vi "Load State.vi"(8 "error in":errorcluster, 11 "State File Refnum":refnum<file>) -> (0 "error out":errorcluster, 1 "Out-of-range List":string[](array[string]), 2 "Monitoring List":string[](array[string]), 3 "refnum out":refnum<file>)   [LabVIEW 2013, in "ACNET Monitor.lvlib"]
uses:
  ACNET Monitor.lvlib
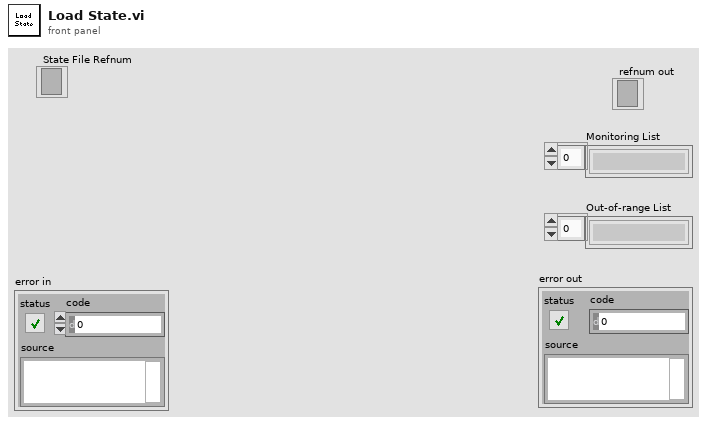
[diagram p1: front panel]
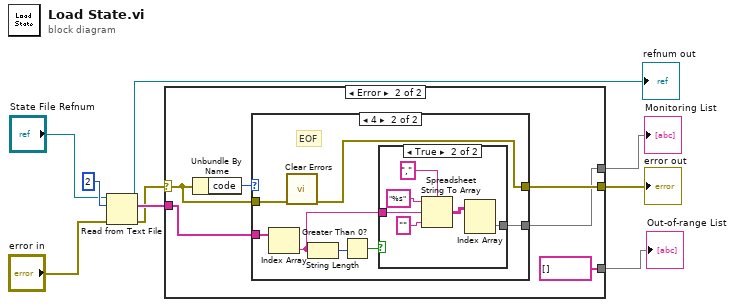
[diagram p0: block diagram]
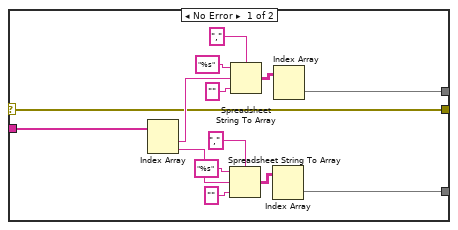
[diagram p2: hidden frame]
diagram:
  n1 = Read from Text File(file (use dialog)="State File Refnum", count=2, error in="error in") -> (refnum out=→"refnum out":refnum<file>, text=w8:string[], error out=w1:errorcluster)  [unwired: 1 in, 1 out]
  n2 = case shown="Error" w1 {
    selector: w1 -> [w12 w28]
    tunnel: w8 -> [w23 w25]
    tunnel: [w12 w27] -> w7
    tunnel: [w11 string[] []] -> w5
    tunnel: [w10 w24] -> w4
    frame No Error {
      n3 = Index Array(array=w23) -> (element #1=w20:string, element #2=w15:string)  [unwired: 2 in]
      n4 = Spreadsheet String To Array(delimiter (Tab)=",", format string="%s", spreadsheet string=w15, array type (2D Dbl)="" ("element")) -> (array=w13:string[][])
      n5 = Spreadsheet String To Array(delimiter (Tab)=",", format string="%s", spreadsheet string=w20, array type (2D Dbl)="" ("element")) -> (array=w14:string[][])
      n6 = Index Array(array=w13) -> (element=w11:string[])  [unwired: 2 in]
      n7 = Index Array(array=w14) -> (element=w10:string[])  [unwired: 2 in]
    }
    frame Error {
      n8 = Unbundle By Name(w28) -> ("code"=w29:i32)
      n9 = case shown="4" w29 {
        tunnel: w28 -> [w30 w37]
        tunnel: [w30 w36] -> w27
        tunnel: w25 -> [_ w35]
        tunnel: [_ w32] -> w24
        frame Default {
        }
        frame 4 {
          # "EOF"
          n10 = Index Array(array=w35) -> (element=w31:string)  [unwired: 1 in]
          n11 = call <vilib>:"Clear Errors.vi"("error in (no error)"=w37) -> ("error out"=w36:errorcluster)  [unwired: 6 in]
          n12 = String Length(string=w31) -> (length=w34:i32)
          n13 = Greater Than 0?(x=w34) -> (x > 0?=w33:bool)
          n14 = case shown="True" w33 {
            tunnel: [_ w39] -> w32
            tunnel: w31 -> [_ w38]
            frame False {
            }
            frame True {
              n15 = Spreadsheet String To Array(delimiter (Tab)=",", format string="%s", spreadsheet string=w38, array type (2D Dbl)="" ("element")) -> (array=w40:string[][])
              n16 = Index Array(array=w40) -> (element=w39:string[])  [unwired: 2 in]
            }
          }
        }
      }
    }
  }
  "error out" <- w7
  "Monitoring List" <- w4
  "Out-of-range List" <- w5
